vi "LWXPS_GPIOAnalogSet.vi"(8 "LabVIEW error IN":errorcluster, 9 "Analog Output Value IN":dbl[](array[numeric]), 10 "GPIO Name IN":string[](array[string]), 11 "XPS Reference IN":refnum<k24>) -> (0 "XPS Error String":string, 1 "Analog Output Value OUT":dbl[](array[numeric]), 2 "GPIO Name OUT":string[](array[string]), 3 "Returned error code":i32, 4 "LabVIEW error OUT":errorcluster, 5 "XPS Reference OUT":refnum<k24>)   [LabVIEW 2014]
uses:
  D:/XPSQ8_LabView_Library/Development/Source/Dll/Newport.XPS.CommandInterface.dll
  Dll/Newport.XPS.CommandInterface.dll
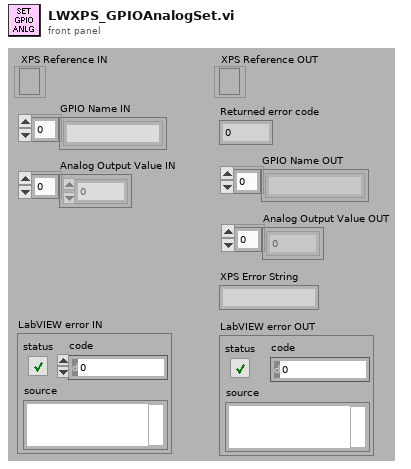
[diagram p1: front panel]
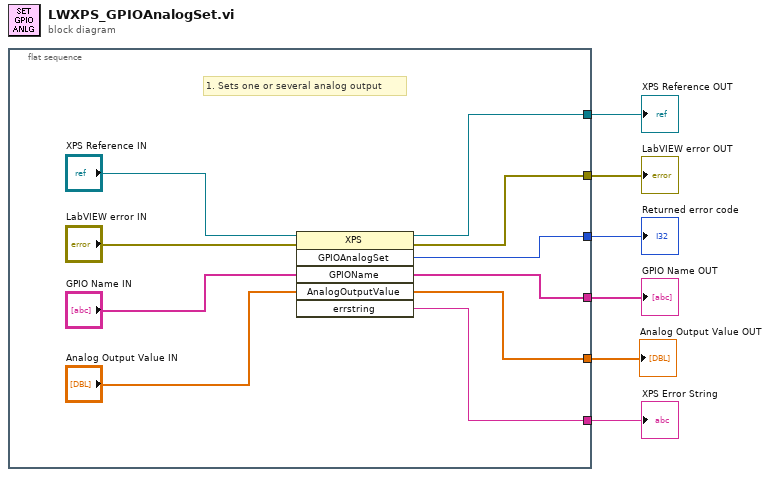
[diagram p0: block diagram]
diagram:
  n1 = flat-sequence {
    tunnel: [w12] -> w6
    tunnel: [w15] -> w5
    tunnel: [w13] -> w4
    tunnel: [w10] -> w1
    tunnel: [w11] -> w2
    tunnel: [w9] -> w3
    frame #0 {
      # "1. Sets one or several analog output"
      n2 = invoke class="XPS" method="GPIOAnalogSet"(reference="XPS Reference IN", error in="LabVIEW error IN", "GPIOName"="GPIO Name IN", "AnalogOutputValue"="Analog Output Value IN") -> (reference out=w12:refnum<k24>, error out=w15:errorcluster, "GPIOAnalogSet"=w13:i32, "GPIOName"=w11:string[], "AnalogOutputValue"=w10:dbl[], "errstring"=w9:string)  [unwired: 2 in]
    }
  }
  "XPS Reference OUT" <- w6
  "LabVIEW error OUT" <- w5
  "Returned error code" <- w4
  "XPS Error String" <- w3
  "GPIO Name OUT" <- w2
  "Analog Output Value OUT" <- w1
